vi "Common_Socket_FWUgrade_Cmd_Sub_VI.vi"(0 "Socket IP Address":string="192.168.1.100", 1 "Response ID 1":u8, 9 "FW Message ID":i32, 11 "FW Message Length":i32, 14 "Time Delay":i16=10) -> (4 "connection ID":refnum<k5>, 6 "Data Response":string, 10 "error out":errorcluster, 15 "Pass":string="Horn Scan Success")   [LabVIEW 2017]
panel:
  in  "error in (no error)":errorcluster
  in  "Socket Port Numeber":u16=1600
  out "*(type *) &x":u8
  out "rest of the binary string":string
  out "Message Length":u8
  out "Message ID":u8
  out "bytes written":i32
  # "Refrence:"
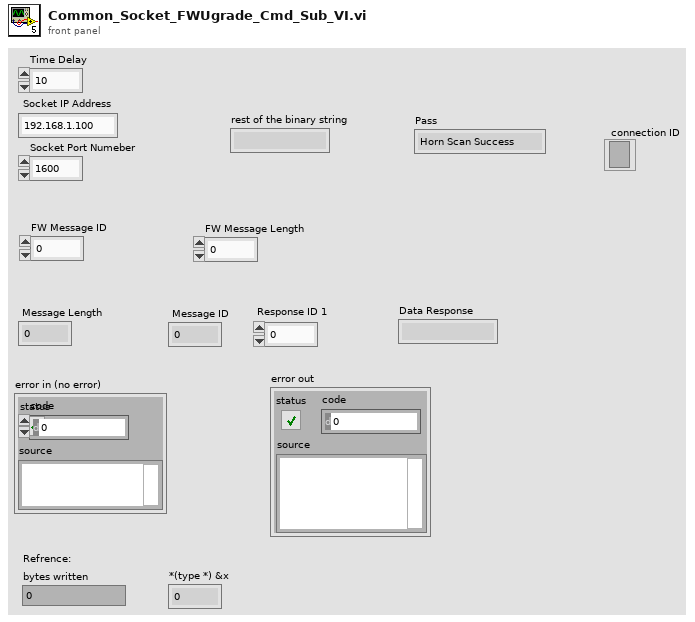
[diagram p1: front panel]
types:
  T1 = enum16{"big-endian, network order", "native, host order", "little-endian"}
  T2 = cluster{"FW Message Length":i32, "FW Message ID":i32}
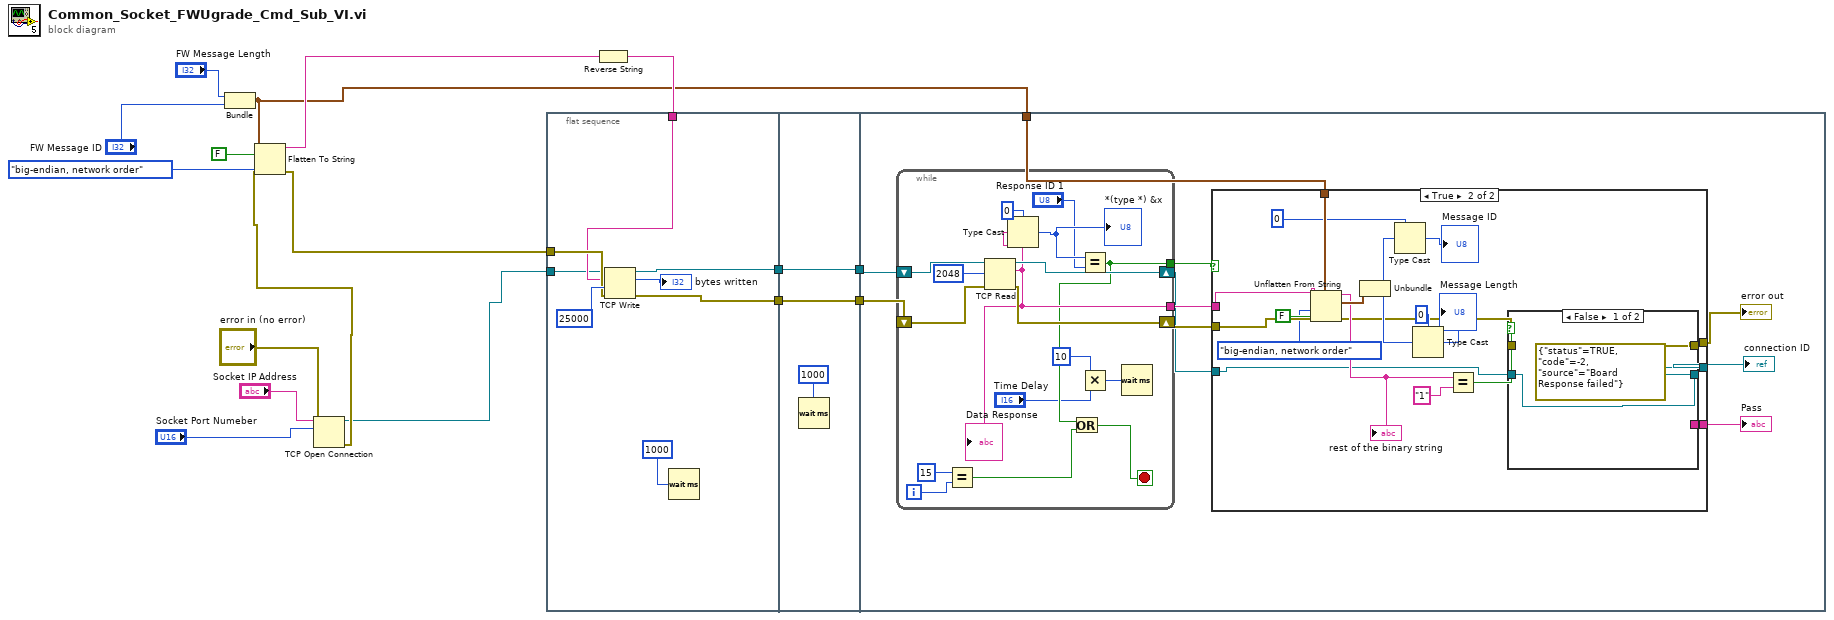
[diagram p0: block diagram]
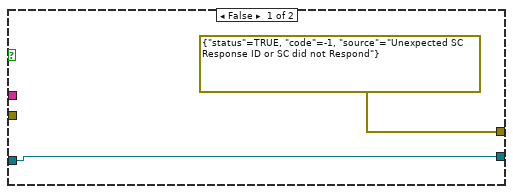
[diagram p2: hidden frame]
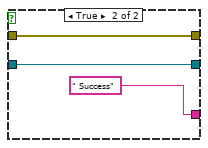
[diagram p3: hidden frame]
diagram:
  n1 = Bundle("FW Message Length"="FW Message Length", "FW Message ID"="FW Message ID") -> (w6:T2)  [unwired: 1 in]
  n2 = TCP Open Connection(address="Socket IP Address", remote port or service name="Socket Port Numeber", error in (no error)="error in (no error)") -> (connection ID=w1:refnum<k5>, error out=w2:errorcluster)  [unwired: 2 in]
  n3 = Flatten To String(anything=w6, prepend array or string size? (T)=FALSE, byte order (0:big-endian, network order)=T1."big-endian, network order", error in (no error)=w2) -> (data string=w9:string, error out=w10:errorcluster)  [unwired: 1 out]
  n4 = flat-sequence {
    tunnel: [w23] -> w17
    tunnel: [w22] -> w16
    tunnel: w10 -> [w21]
    tunnel: w8 -> [w20]
    tunnel: w1 -> [w18]
    tunnel: [w27] -> w15
    tunnel: w17 -> [w27]
    tunnel: [w26] -> w14
    tunnel: w16 -> [w26]
    tunnel: w15 -> [w38]
    tunnel: w14 -> [w37]
    tunnel: w6 -> [w36]
    frame #0 {
      n5 = TCP Write(connection ID=w18, data in=w20, error in (no error)=w21, 9:25000 ("timeout ms (25000)")) -> (connection ID out=w23:refnum<k5>, bytes written=→"bytes written":i32, error out=w22:errorcluster)
      n6 = Wait (ms)(milliseconds to wait=u32 1000) -> ()  [unwired: 1 out]
    }
    frame #1 {
      n7 = Wait (ms)(milliseconds to wait=u32 1000) -> ()  [unwired: 1 out]
    }
    frame #2 {
      n8 = while {
        tunnel: [w77] -> w35
        shift-right: [w80] -> w31
        shift-left: w38 -> [w82]
        shift-right: [w78] -> w34
        shift-left: w37 -> [w81]
        tunnel: [w73] -> w33
        i -> [w71]
        stop <- w72 stop-if-true
        n9 = Equal?(x=15, y=w71) -> (x = y?=w69:bool)
        n10 = TCP Read(connection ID=w82, bytes to read=2048, error in (no error)=w81) -> (connection ID out=w80:refnum<k5>, data out=w77:string, error out=w78:errorcluster)  [unwired: 2 in]
        "Data Response" <- w77
        n11 = Type Cast(type=u8 0, x=w77) -> (*(type *) &x=w75:u8)
        "*(type *) &x" <- w75
        n12 = Equal?(x=w75, y="Response ID 1") -> (x = y?=w73:bool)
        n13 = Or(x=w73, y=w69) -> (x .or. y?=w72:bool)
        n14 = Multiply(x=i16 10 ("milliseconds to wait"), y="Time Delay") -> (x*y=w67:i16)
        n15 = Wait (ms)(milliseconds to wait=w67) -> ()  [unwired: 1 out]
      }
      n16 = case shown="True" w33 {
        tunnel: w36 -> [_ w59]
        tunnel: w35 -> [_ w51]
        tunnel: w34 -> [_ w50]
        tunnel: [w40 w42] -> w32
        tunnel: w31 -> [w40 w43]
        tunnel: [errorcluster {"status"=TRUE, "code"=-1, "source"="Unexpected SC Response ID or SC did not Respond"} ("error constant") w44] -> w30
        tunnel: [_ w41] -> w29
        frame False {
        }
        frame True {
          n17 = Unflatten From String(type=w59, binary string=w51, data includes array or string size? (T)=FALSE, byte order (0:big-endian, network order)=T1."big-endian, network order", error in (no error)=w50) -> (rest of the binary string=w48:string, value=w60:T2, error out=w45:errorcluster)
          "rest of the binary string" <- w48
          n18 = Unbundle(w60) -> ("FW Message Length"=w53:i32, "FW Message ID"=w57:i32)
          n19 = Type Cast(type=u8 0, x=w53) -> (*(type *) &x=→"Message ID":u8)
          n20 = Type Cast(type=u8 0, x=w57) -> (*(type *) &x=→"Message Length":u8)
          n21 = Equal?(x=w48, y="1") -> (x = y?=w46:bool)
          n22 = case shown="False" w46 {
            tunnel: w45 -> [_ w65]
            tunnel: [errorcluster {"status"=TRUE, "code"=-2, "source"="Board Response failed"} ("error constant") w65] -> w44
            tunnel: w43 -> [w61 w64]
            tunnel: [w61 w64] -> w42
            tunnel: [_ " Success"] -> w41
            frame False {
            }
            frame True {
            }
          }
        }
      }
      "error out" <- w30
      "connection ID" <- w32
      "Pass" <- w29
    }
  }
  n23 = Reverse String(1:w9) -> (0:w8:string)
